vi "Initialize Device Core.vi"(8 "error in (no error)":errorcluster, 9 "Reset (F)":bool, 10 "Resource Name":string, 11 "BNT_ULx-MCSV in":refnum<class "BNT_ULx-MCSV.lvclass">) -> (0 "error out":errorcluster, 3 "BNT_ULx-MCSV out":refnum<class "BNT_ULx-MCSV.lvclass">)   [LabVIEW 2020, in "BNT_ULx.lvlib" / "BNT_ULx-MCSV.lvclass"]
doc: "Initialize device driver."
uses:
  BNT_ULx-MCSV.lvclass
  BNT_ULx-MCSV.lvclass/BNT_ULx-MCSV.ctl
  C:/Program Files (x86)/National Instruments/LabVIEW 2020/vi.lib/ULx/ULx_LV.dll
  Program Files (x86)/National Instruments/LabVIEW 2020/vi.lib/ULx/ULx_LV.dll
  CSPP_Core/Actors/CSPP_DeviceActor/CSPP_DeviceActor.lvclass
  <vilib>/ULx/Create Channel.llb/ULx Create Channel (DI-Digital Input).vi
  <vilib>/ULx/Create Channel.llb/ULx Create Channel (DO-Digital Output).vi
  <vilib>/ULx/Read.llb/ULx Read (Analog 1D DBL NChan 1Samp).vi
  <vilib>/ULx/Read.llb/ULx Read (Digital 1D Bool NChan 1Samp 1Line).vi
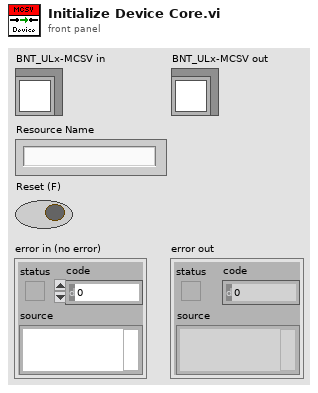
[diagram p1: front panel]
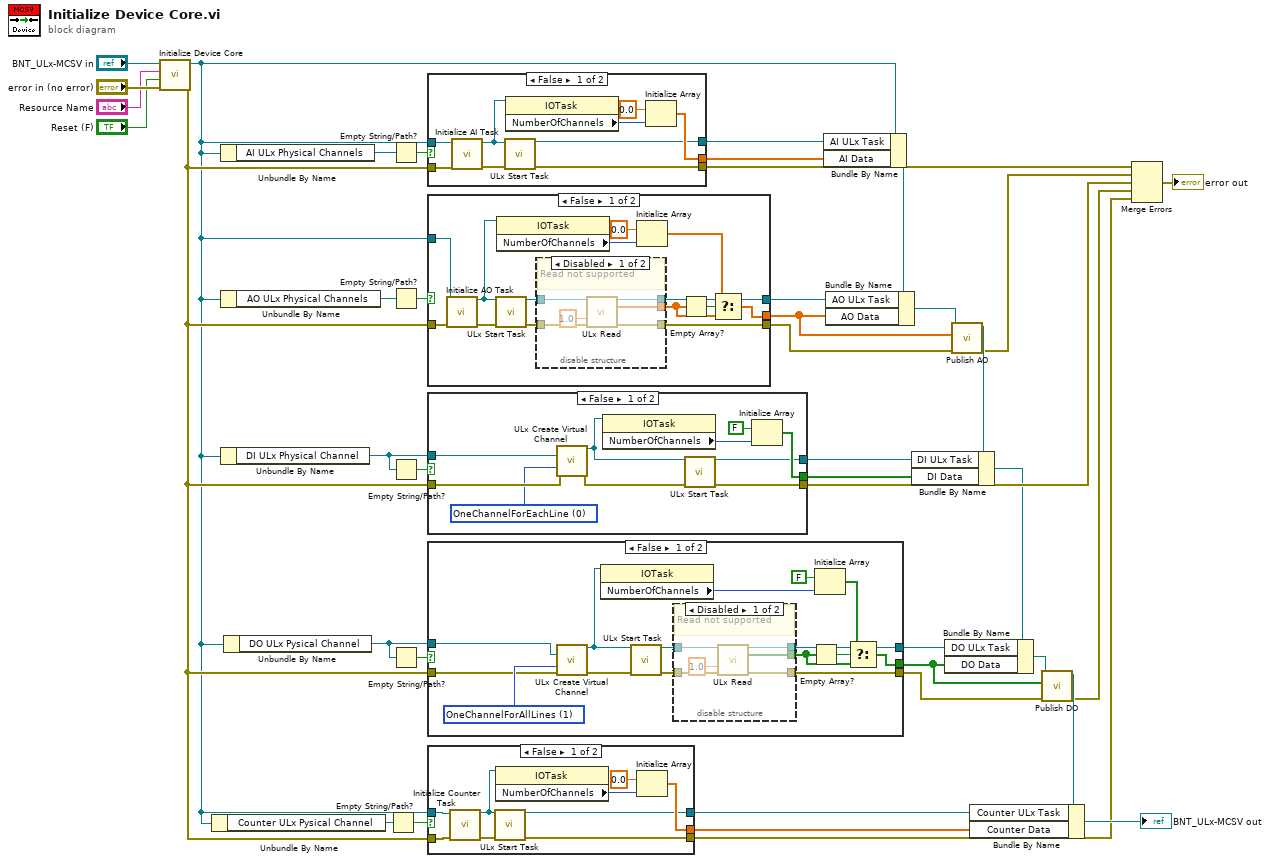
[diagram p0: block diagram]
diagram:
  n1 = call-parent "Initialize Device Core.vi"("error in (no error)"="error in (no error)", "Reset (F)"="Reset (F)", "Resource Name"="Resource Name", "CSPP_DeviceActor in"="BNT_ULx-MCSV in") -> ("error out"=w19:errorcluster, "CSPP_DeviceActor out"=w15:refnum<class "BNT_ULx-MCSV.lvclass">)  [unwired: 6 in]
  n2 = Unbundle By Name(w15) -> ("Counter ULx Pysical Channel"=w20:refnum<k21>)
  n3 = Unbundle By Name(w15) -> ("AI ULx Physical Channels"=w32:refnum<k21>)
  n4 = Unbundle By Name(w15) -> ("AO ULx Physical Channels"=w30:refnum<k21>)
  n5 = Unbundle By Name(w15) -> ("DI ULx Physical Channel"=w27:refnum<k21>)
  n6 = Unbundle By Name(w15) -> ("DO ULx Pysical Channel"=w24:refnum<k21>)
  n7 = Empty String/Path?(string/path=w20) -> (empty?=w21:bool)
  n8 = Empty String/Path?(string/path=w32) -> (empty?=w31:bool)
  n9 = Empty String/Path?(string/path=w30) -> (empty?=w29:bool)
  n10 = Empty String/Path?(string/path=w27) -> (empty?=w28:bool)
  n11 = Empty String/Path?(string/path=w24) -> (empty?=w23:bool)
  n12 = case shown="False" w31 {
    tunnel: [w44 _] -> w37
    tunnel: w19 -> [w49 w51]
    tunnel: [w45 w51] -> w34
    tunnel: w15 -> [w50 _]
    tunnel: [w47 _] -> w14
    frame False {
      n13 = call-dynamic "Initialize AI Task.vi"("error in (no error)"=w49, "BNT_ULx-MCSV in"=w50) -> ("error out"=w46:errorcluster, "AI ULx Task"=w43:refnum<k24>)  [unwired: 8 in]
      n14 = call <vilib>:"ULx Start Task.vi"("task in"=w43, "error in"=w46) -> ("task out"=w44:refnum<k24>, "error out"=w45:errorcluster)  [unwired: 12 in]
      n15 = property class="IOTask"(reference=w43) -> ("NumberOfChannels"=w42:u32)  [unwired: 1 in, 2 out]
      n16 = Initialize Array(0.0 ("element"), w42) -> (w47:dbl[])
    }
    frame True {
    }
  }
  n17 = case shown="False" w29 {
    tunnel: [w53 _] -> w36
    tunnel: w19 -> [w65 w74]
    tunnel: [w55 w74] -> w10
    tunnel: [w60 _] -> w9
    tunnel: w15 -> [w64 _]
    frame False {
      n18 = call-dynamic "Initialize AO Task.vi"("error in (no error)"=w65, "BNT_ULx-MCSV in"=w64) -> ("error out"=w59:errorcluster, "AO ULx Task"=w58:refnum<k24>)  [unwired: 8 in]
      n19 = call <vilib>:"ULx Start Task.vi"("task in"=w58, "error in"=w59) -> ("task out"=w54:refnum<k24>, "error out"=w56:errorcluster)  [unwired: 12 in]
      n20 = property class="IOTask"(reference=w58) -> ("NumberOfChannels"=w57:u32)  [unwired: 1 in, 2 out]
      n21 = disable-structure shown="Disabled" {
        disable-tunnel: w56 -> [w71 w72]
        disable-tunnel: [w70 w72] -> w55
        disable-tunnel: w54 -> [w69 w73]
        disable-tunnel: [w68 w73] -> w53
        disable-tunnel: [w67 _] -> w52
        frame Disabled {
          # "Read not supported"
          n22 = call-poly <vilib>:"ULx Read.vi"("task in"=w69, "timeout"=1.0, "error in"=w71) -> ("task out"=w68:refnum<k24>, "data"=w67:dbl[], "error out"=w70:errorcluster)  [unwired: 10 in]
        }
        frame Enabled {
        }
      }
      n23 = Initialize Array(0.0 ("element"), w57) -> (w61:dbl[])
      n24 = Empty Array?(array=w52) -> (empty?=w62:bool)
      n25 = Select(t=w61, s=w62, f=w52) -> (s? t:f=w60:dbl[])
    }
    frame True {
    }
  }
  n26 = case shown="False" w28 {
    tunnel: [w81 _] -> w26
    tunnel: [w82 w85] -> w25
    tunnel: w19 -> [w78 w85]
    tunnel: w27 -> [w80 _]
    tunnel: [w83 _] -> w8
    frame False {
      w75 = 0 items=["OneChannelForEachLine", "OneChannelForAllLines"] ("line grouping")
      n27 = call-poly <vilib>:"ULx Create Virtual Channel.vi"("lines"=w80, "line grouping"=w75, "error in"=w78) -> ("task out"=w77:refnum<k24>, "error out"=w79:errorcluster)  [unwired: 11 in]
      n28 = property class="IOTask"(reference=w77) -> ("NumberOfChannels"=w76:u32)  [unwired: 1 in, 2 out]
      n29 = call <vilib>:"ULx Start Task.vi"("task in"=w77, "error in"=w79) -> ("task out"=w81:refnum<k24>, "error out"=w82:errorcluster)  [unwired: 12 in]
      n30 = Initialize Array(FALSE, w76) -> (w83:bool[])
    }
    frame True {
    }
  }
  n31 = case shown="False" w23 {
    tunnel: [w88 _] -> w1
    tunnel: [w90 w109] -> w5
    tunnel: w19 -> [w86 w109]
    tunnel: w24 -> [w94 _]
    tunnel: [w97 _] -> w3
    frame False {
      w95 = 1 items=["OneChannelForEachLine", "OneChannelForAllLines"] ("line grouping")
      n32 = call-poly <vilib>:"ULx Create Virtual Channel.vi"("lines"=w94, "line grouping"=w95, "error in"=w86) -> ("task out"=w93:refnum<k24>, "error out"=w96:errorcluster)  [unwired: 11 in]
      n33 = property class="IOTask"(reference=w93) -> ("NumberOfChannels"=w92:u32)  [unwired: 1 in, 2 out]
      n34 = call <vilib>:"ULx Start Task.vi"("task in"=w93, "error in"=w96) -> ("task out"=w89:refnum<k24>, "error out"=w91:errorcluster)  [unwired: 12 in]
      n35 = disable-structure shown="Disabled" {
        disable-tunnel: w91 -> [w106 w107]
        disable-tunnel: [w105 w107] -> w90
        disable-tunnel: w89 -> [w103 w108]
        disable-tunnel: [w102 w108] -> w88
        disable-tunnel: [w101 _] -> w87
        frame Disabled {
          # "Read not supported"
          n36 = call-poly <vilib>:"ULx Read.vi"("task in"=w103, "timeout"=1.0, "error in"=w106) -> ("task out"=w102:refnum<k24>, "data"=w101:bool[], "error out"=w105:errorcluster)  [unwired: 10 in]
        }
        frame Enabled {
        }
      }
      n37 = Empty Array?(array=w87) -> (empty?=w99:bool)
      n38 = Initialize Array(FALSE, w92) -> (w98:bool[])
      n39 = Select(t=w98, s=w99, f=w87) -> (s? t:f=w97:bool[])
    }
    frame True {
    }
  }
  n40 = case shown="False" w21 {
    tunnel: [w112 _] -> w18
    tunnel: w19 -> [w117 w119]
    tunnel: [w113 w119] -> w16
    tunnel: w15 -> [w118 _]
    tunnel: [w115 _] -> w2
    frame False {
      n41 = call-dynamic "Initialize Counter Task.vi"("error in (no error)"=w117, "BNT_ULx-MCSV in"=w118) -> ("error out"=w114:errorcluster, "Counter ULx Task"=w111:refnum<k24>)  [unwired: 8 in]
      n42 = call <vilib>:"ULx Start Task.vi"("task in"=w111, "error in"=w114) -> ("task out"=w112:refnum<k24>, "error out"=w113:errorcluster)  [unwired: 12 in]
      n43 = property class="IOTask"(reference=w111) -> ("NumberOfChannels"=w110:u32)  [unwired: 1 in, 2 out]
      n44 = Initialize Array(0.0, w110) -> (w115:dbl[])
    }
    frame True {
    }
  }
  n45 = Bundle By Name(cluster=w15, "AI ULx Task"=w37, "AI Data"=w14) -> (w35:refnum<class "BNT_ULx-MCSV.lvclass">)
  n46 = Bundle By Name(cluster=w35, "AO ULx Task"=w36, "AO Data"=w9) -> (w13:refnum<class "BNT_ULx-MCSV.lvclass">)
  n47 = call "Publish AO.vi"("error in"=w10, "AO Data"=w9, "BNT_ULx-MCSV in"=w13) -> ("error out"=w11:errorcluster, "BNT_ULx-MCSV out"=w12:refnum<class "BNT_ULx-MCSV.lvclass">)  [unwired: 7 in]
  n48 = Bundle By Name(cluster=w12, "DI ULx Task"=w26, "DI Data"=w8) -> (w22:refnum<class "BNT_ULx-MCSV.lvclass">)
  n49 = Bundle By Name(cluster=w22, "DO ULx Task"=w1, "DO Data"=w3) -> (w7:refnum<class "BNT_ULx-MCSV.lvclass">)
  n50 = call "Publish DO.vi"("error in"=w5, "DO Data"=w3, "BNT_ULx-MCSV in"=w7) -> ("error out"=w4:errorcluster, "BNT_ULx-MCSV out"=w6:refnum<class "BNT_ULx-MCSV.lvclass">)  [unwired: 7 in]
  n51 = Bundle By Name(cluster=w6, "Counter ULx Task"=w18, "Counter Data"=w2) -> (→"BNT_ULx-MCSV out":refnum<class "BNT_ULx-MCSV.lvclass">)
  n52 = Merge Errors(w34, w11, w25, w4, w16) -> (→"error out":errorcluster)
